vi "get3Ddata.vi"(9 "plottedVariables":i32[](array[numeric]), 10 "Plotted Series":bool[][](array[boolean]), 11 "allTheData":string[][](array[string])) -> (1 "scalarVals":dbl[](array[numeric]), 3 "vectorInfo":T2 {"UVW-TI" format="%#_3g"; "XYZ-WD" format="%#_3g"}, 4 "STLs":cluster{"coordSys":T1, "WD":dbl, "STL":string}[](array[cluster]), 5 "mostCoords":T1)   [LabVIEW 2022 SP3]
uses:
  vectorDef.ctl
  coordSys.ctl
  <vilib>/Analysis/baseanly.llb/Mean (DBL).vi
  e7cd0213-2e99-7242-882f-f13518424f13.vi
  Anemometry/Anemometry Sub Vis/Data_plotting_vis/Results_plotter_Global.vi
  <vilib>/Analysis/NI_AALBase.lvlib
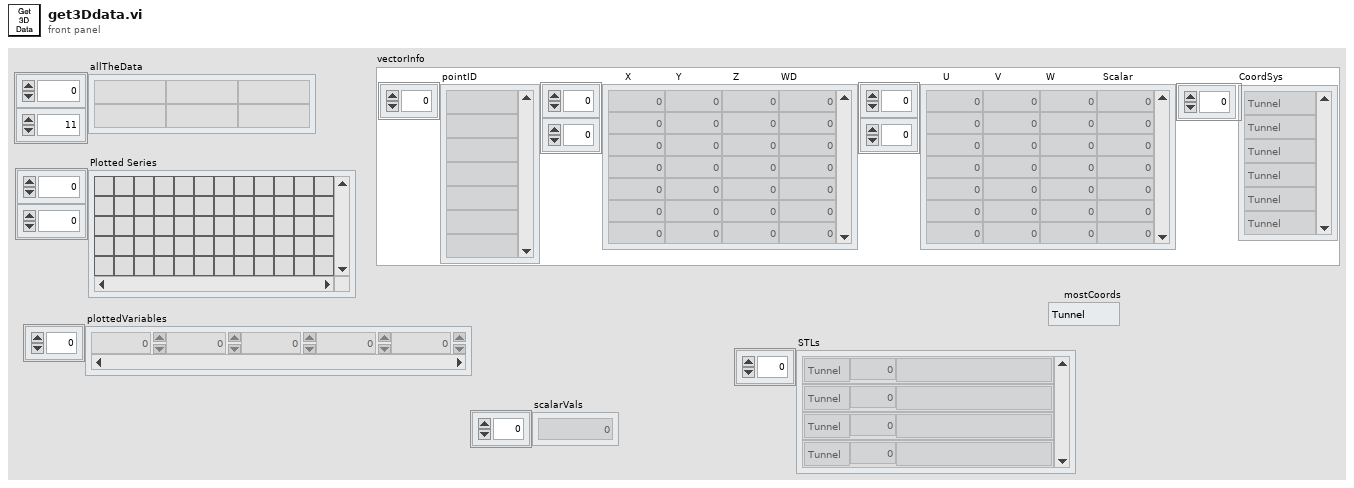
[diagram p1: front panel]
types:
  T1 = typedef "coordSys.ctl" = enum16{"Tunnel", "Model"}
  T2 = typedef "vectorDef.ctl" = cluster{"pointID":string[], "XYZ-WD":dbl[][], "UVW-TI":dbl[][], "CoordSys":T1[]}
  T3 = cluster{"Enum":T1, "Numeric":dbl, "String Out":string}[]
  T4 = cluster{"Enum":T1, "Numeric":dbl, "String Out":string}
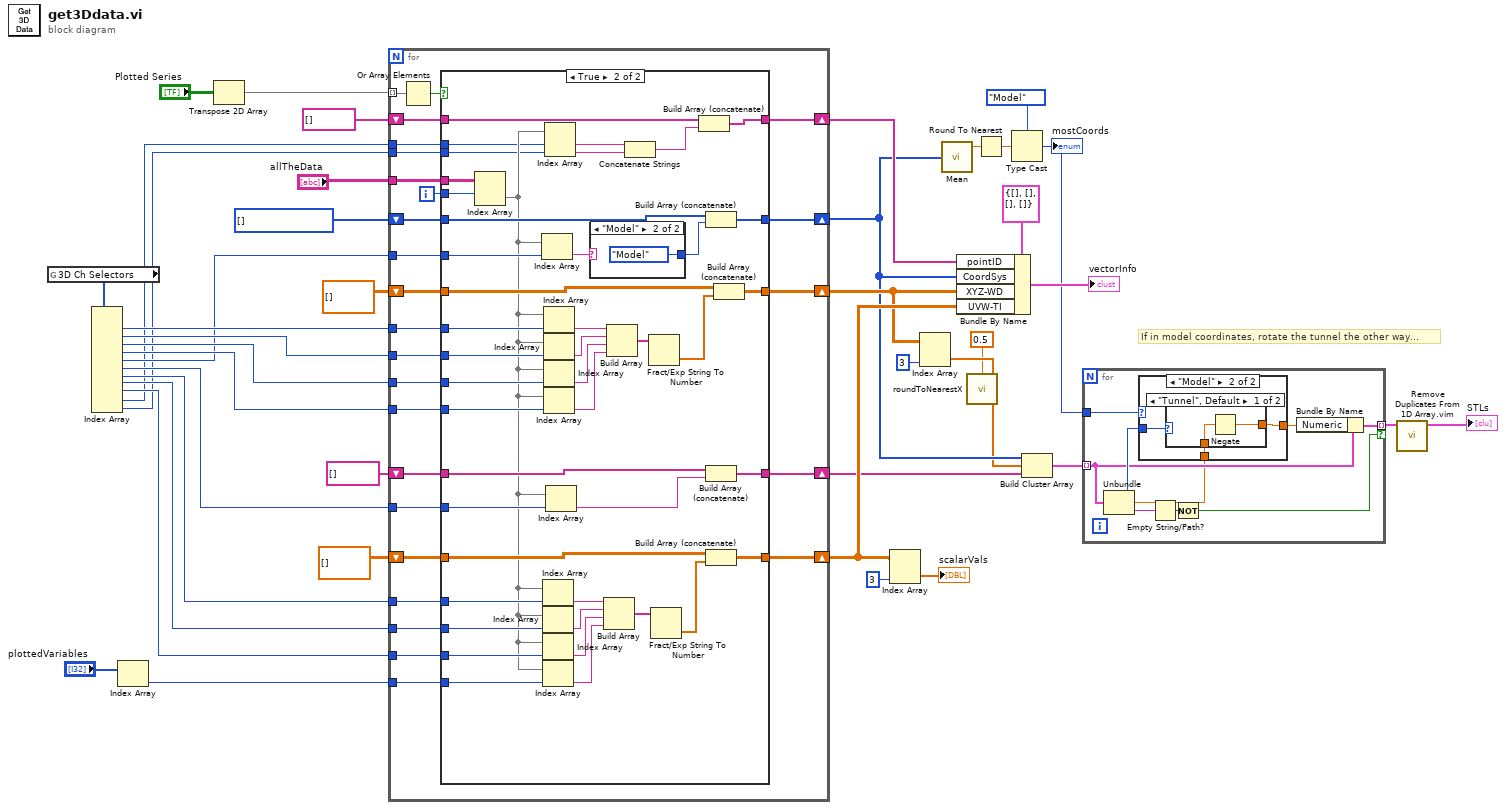
[diagram p0: block diagram]
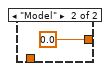
[diagram p3: hidden frame]
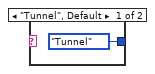
[diagram p5: hidden frame]
diagram:
  w16 = T1[] [] items=["Tunnel", "Model"]
  # "If in model coordinates, rotate the tunnel the other way..."
  n1 = global read "Results_plotter_Global.vi" "3D Ch Selectors"() -> (w41:i32[])
  n2 = Index Array(array=w41) -> (element #1=w37:i32, element #2=w36:i32, element #3=w35:i32, element #4=w34:i32, element #5=w33:i32, element #6=w32:i32, element #7=w31:i32, element #8=w30:i32, element #9=w29:i32, element #10=w3:i32, element #11=w1:i32)  [unwired: 11 in]
  n3 = Index Array(array="plottedVariables") -> (element=w28:i32)  [unwired: 1 in]
  n4 = Transpose 2D Array(2D array="Plotted Series") -> (transposed array=w19:bool[][])
  n5 = for {
    tunnel: w19 -> [w68] mode=indexing
    tunnel: "allTheData" -> [w67]
    tunnel: w37 -> [w65]
    tunnel: w36 -> [w64]
    tunnel: w35 -> [w63]
    tunnel: w34 -> [w62]
    tunnel: w33 -> [w61]
    tunnel: w32 -> [w60]
    tunnel: w31 -> [w59]
    tunnel: w30 -> [w58]
    tunnel: w29 -> [w57]
    tunnel: w28 -> [w56]
    shift-right: [w54] -> w17
    shift-left: dbl[][] [] -> [w55]
    shift-right: [w53] -> w27
    shift-left: string[] [] -> [w52]
    shift-right: [w51] -> w24
    shift-left: dbl[][] [] -> [w50]
    shift-right: [w48] -> w11
    shift-left: string[] [] -> [w49]
    shift-right: [w46] -> w12
    shift-left: w16 -> [w45]
    tunnel: w3 -> [w44]
    tunnel: w1 -> [w43]
    i -> [w66]
    n6 = Or Array Elements(Boolean array=w68) -> (logical OR=w47:bool)
    n7 = case shown="True" w47 {
      tunnel: w67 -> [_ w116]
      tunnel: w66 -> [_ w78]
      tunnel: w65 -> [_ w115]
      tunnel: w64 -> [_ w114]
      tunnel: w63 -> [_ w113]
      tunnel: w62 -> [_ w112]
      tunnel: w61 -> [_ w111]
      tunnel: w60 -> [_ w110]
      tunnel: w59 -> [_ w109]
      tunnel: w58 -> [_ w108]
      tunnel: w57 -> [_ w107]
      tunnel: w56 -> [_ w106]
      tunnel: w55 -> [w73 w99]
      tunnel: [w73 w98] -> w54
      tunnel: [w72 w97] -> w53
      tunnel: w52 -> [w72 w96]
      tunnel: w50 -> [w71 w89]
      tunnel: [w71 w90] -> w51
      tunnel: w49 -> [w70 w87]
      tunnel: [w70 w86] -> w48
      tunnel: [w69 w84] -> w46
      tunnel: w45 -> [w69 w83]
      tunnel: w44 -> [_ w79]
      tunnel: w43 -> [_ w75]
      frame False {
      }
      frame True {
        n8 = Index Array(array=w116, index (row)=w78) -> (element=w80:string[])  [unwired: 1 in]
        n9 = Index Array(array=w80, index=w111) -> (element=w82:string)
        n10 = Index Array(array=w80, index=w109) -> (element=w94:string)
        n11 = Index Array(array=w80, index=w108) -> (element=w93:string)
        n12 = Index Array(array=w80, index=w107) -> (element=w92:string)
        n13 = Index Array(array=w80, index=w106) -> (element=w91:string)
        n14 = Index Array(array=w80, index=w115) -> (element=w105:string)
        n15 = Index Array(array=w80, index=w114) -> (element=w104:string)
        n16 = Index Array(array=w80, index=w113) -> (element=w103:string)
        n17 = Index Array(array=w80, index=w112) -> (element=w102:string)
        n18 = Index Array(array=w80, index #1=w79, index #2=w75) -> (element #1=w77:string, element #2=w74:string)
        n19 = Index Array(array=w80, index=w110) -> (element=w85:string)
        n20 = case shown="\"Model\"" w82 {
          tunnel: [coordSys."Tunnel" ("Enum") coordSys."Model" ("Enum")] -> w81
          frame "Tunnel", Default {
          }
          frame "Model" {
          }
        }
        n21 = Build Array(w94, w93, w92, w91) -> (w95:string[])
        n22 = Build Array(w105, w104, w103, w102) -> (w101:string[])
        n23 = Concatenate Strings(w77, w74) -> (w76:string)
        n24 = Fract/Exp String To Number(string=w101) -> (number=w100:dbl[])  [unwired: 3 in, 1 out]
        n25 = Fract/Exp String To Number(string=w95) -> (number=w88:dbl[])  [unwired: 3 in, 1 out]
        n26 = Build Array (concatenate)(w96, w76) -> (w97:string[])
        n27 = Build Array (concatenate)(w83, w81) -> (w84:T1[])
        n28 = Build Array (concatenate)(w87, w85) -> (w86:string[])
        n29 = Build Array (concatenate)(w89, w88) -> (w90:dbl[][])
        n30 = Build Array (concatenate)(w99, w100) -> (w98:dbl[][])
      }
    }
  }
  n31 = Index Array(array=w24, index (col)=3 ("disabled index (col)")) -> (element=→"scalarVals":dbl[])  [unwired: 1 in]
  n32 = Index Array(array=w17, index (col)=3 ("disabled index (col)")) -> (element=w10:dbl[])  [unwired: 1 in]
  n33 = call-poly <vilib>:"Mean.vi"("X"=w12) -> ("mean"=w15:dbl)  [unwired: 1 out]
  n34 = Bundle By Name(cluster=T2 {"pointID"=[], "XYZ-WD"=[], "UVW-TI"=[], "CoordSys"=[]} ("vectorInfo"), "pointID"=w27, "CoordSys"=w12, "XYZ-WD"=w17, "UVW-TI"=w24) -> (→"vectorInfo":T2)
  n35 = call "roundToNearestX.vi"("Round to Nearest"=0.5, "Array"=w10) -> ("roundedArray"=w9:dbl[])  [unwired: 1 in, 1 out]
  n36 = Round To Nearest(number=w15) -> (nearest integer value=w14:dbl)
  n37 = Type Cast(type=coordSys."Model" ("Enum"), x=w14) -> (*(type *) &x=w7:T1)
  "mostCoords" <- w7
  n38 = Build Cluster Array(w12, w9, w11) -> (w6:T3)
  n39 = for {
    tunnel: w6 -> [w122] mode=indexing
    tunnel: [w121] -> w5 mode=indexing if=w125
    tunnel: w7 -> [w124]
    n40 = Unbundle(w122) -> ("Enum"=w123:T1, "Numeric"=w119:dbl, "String Out"=w127:string)
    n41 = case shown="\"Model\"" w124 {
      tunnel: w123 -> [_ w130]
      tunnel: [w128 w131] -> w120
      tunnel: w119 -> [w128 w129]
      frame "Tunnel", Default {
      }
      frame "Model" {
        n42 = case shown="\"Tunnel\", Default" w130 {
          tunnel: [w132 0.0 ("Numeric")] -> w131
          tunnel: w129 -> [w133 _]
          frame "Tunnel", Default {
            n43 = Negate(x=w133) -> (-x=w132:dbl)
          }
          frame "Model" {
          }
        }
      }
    }
    n44 = Empty String/Path?(string/path=w127) -> (empty?=w126:bool)
    n45 = Not(x=w126) -> (.not. x?=w125:bool)
    n46 = Bundle By Name(cluster=w122, "Numeric"=w120) -> (w121:T4)
  }
  n47 = call "Remove Duplicates From 1D Array.vim"("array"=w5) -> ("array with duplicates removed"=→"STLs":T3)  [unwired: 10 in]
